vi "Configure RTD [RTD] Core.vi"(8 "error in (no error)":errorcluster, 9 "resistance (0.0 ohms)":dbl format="%^.2e", 10 "alpha (0.0)":dbl format="%^.2e", 11 "CS++DMM in":refnum<class "CS++DMM.lvclass">) -> (0 "error out":errorcluster, 3 "CS++DMM out":refnum<class "CS++DMM.lvclass">)   [LabVIEW 2016, in "CS++DMM.lvlib" / "CS++DMM.lvclass"]
doc: "This VI configures the alpha and resistance parameters for a resistance temperature device.\n\nThis VI affects the behavior of the instrument only when the IviDmm>Temperature Measurements>Transducer Type [TMP] property is set to IVIDMM_VAL_2_WIRE_RTD or IVIDMM_VAL_4_WIRE_RTD.\n\nNote:\n\n(1) This VI is part of the IviDmmResistanceTemperatureDevice [RTD] extension group.\n\n(2) The driver assumes that you are using a Platinum Resistance Temperature Device."
uses:
  CS++DMM.lvclass
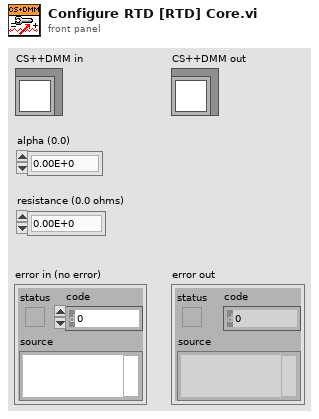
[diagram p1: front panel]
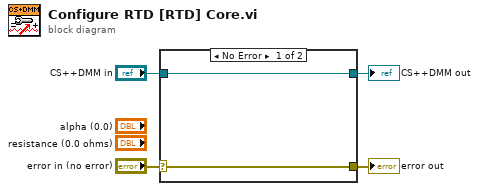
[diagram p0: block diagram]
diagram:
  n1 = case shown="No Error" "error in (no error)" {
    selector: "error in (no error)" -> [w5 w8]
    tunnel: [w5 w8] -> w3
    tunnel: [w6 w7] -> w1
    tunnel: "CS++DMM in" -> [w6 w7]
    frame No Error {
    }
    frame Error {
    }
  }
  "error out" <- w3
  "CS++DMM out" <- w1
